vi "DetectorReadData-nil.vi"(8 "error in (no error)":errorcluster, 9 "disable averaging":bool, 10 "show flyback data":bool, 11 "Microscope in":refnum<class "Microscope.lvclass">) -> (0 "error out":errorcluster, 2 "Data":dbl[][](array[numeric]), 3 "Microscope out":refnum<class "Microscope.lvclass">)   [LabVIEW 2012, in "Microscope.lvclass"]
uses:
  classes/Microscope.lvclass
  classes/Microscope.lvclass/Microscope.ctl
  <resource>/objmgr/daqmx.rc
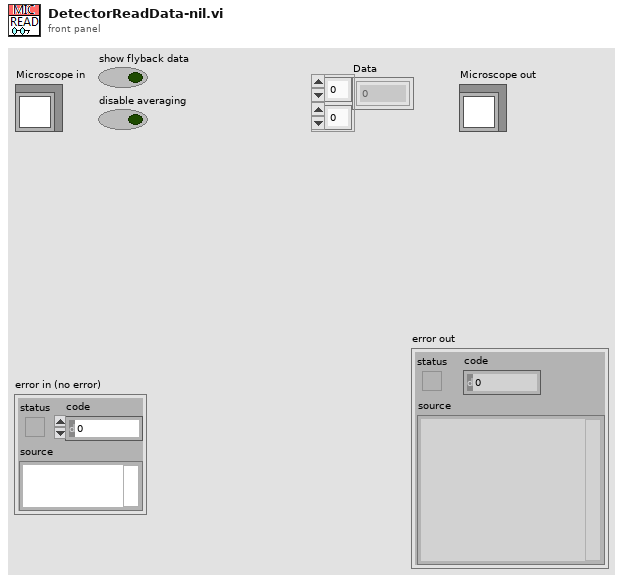
[diagram p1: front panel]
types:
  T1 = typedef "DetectorType.ctl" = enum16{"PMT", "SpectraWiz"}
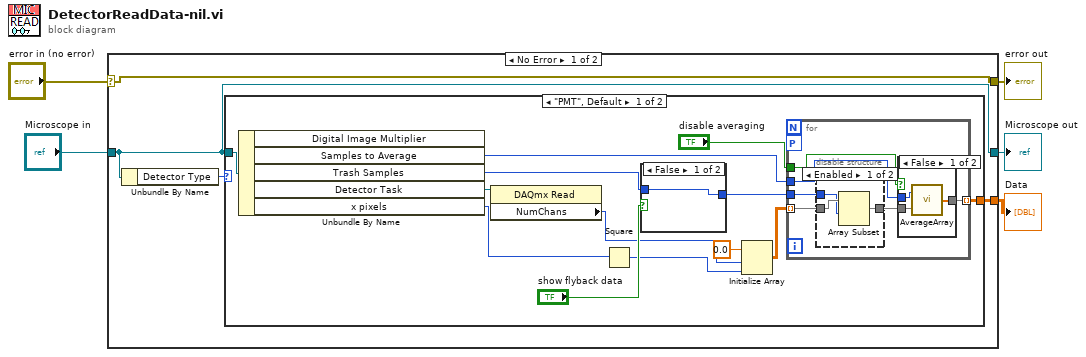
[diagram p0: block diagram]
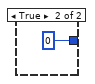
[diagram p2: hidden frame]
diagram:
  n1 = case shown="No Error" "error in (no error)" {
    selector: "error in (no error)" -> [w8 w40]
    tunnel: [w8 w40] -> w4
    tunnel: [w6 w39] -> w2
    tunnel: "Microscope in" -> [w6 w39]
    tunnel: [w9 _] -> w1
    frame No Error {
      n2 = Unbundle By Name(w6) -> ("Detector Type"=w7:T1)
      n3 = case shown="\"PMT\", Default" w7 {
        tunnel: [w22 _] -> w9
        tunnel: w6 -> [w10 _]
        frame "PMT", Default {
          n4 = Unbundle By Name(w10) -> ("Samples to Average"=w21:i32, "Trash Samples"=w20:i32, "Detector Task"=w15:refnum<k21>, "x pixels"=w13:i32)  [unwired: 1 out]
          n5 = property class="DAQmx Read"(reference=w15) -> ("NumChans"=w14:u32)  [unwired: 1 in, 2 out]
          n6 = Square(x=w13) -> (x^2=w12:i32)
          n7 = case shown="False" "show flyback data" {
            tunnel: w20 -> [w23 _]
            tunnel: [w23 0 ("Trash Samples")] -> w19
            frame False {
            }
            frame True {
            }
          }
          n8 = Initialize Array(0.0 ("element"), w14, w12) -> (w11:dbl[][])
          n9 = for {
            tunnel: w11 -> [w26] mode=indexing
            tunnel: w21 -> [w29]
            tunnel: w19 -> [w27]
            tunnel: [w28] -> w22 mode=indexing
            tunnel: "disable averaging" -> [w25]
            workers-P: _ -> [_]
            n10 = disable-structure shown="Enabled" {
              disable-tunnel: [w37 w38] -> w30
              disable-tunnel: w26 -> [w36 w38]
              disable-tunnel: w27 -> [w35 _]
              frame Enabled {
                n11 = Array Subset(array=w36, index=w35) -> (w37:dbl[])  [unwired: 1 in]
              }
              frame Disabled {
              }
            }
            n12 = case shown="False" w25 {
              tunnel: w30 -> [w33 w34]
              tunnel: w29 -> [w32 _]
              tunnel: [w31 w34] -> w28
              frame False {
                n13 = call "AverageArray.vi"("Input Array"=w33, "Samples To Average"=w32) -> ("Averaged Array"=w31:dbl[])
              }
              frame True {
              }
            }
          }
        }
        frame "SpectraWiz" {
        }
      }
    }
    frame Error {
    }
  }
  "error out" <- w4
  "Microscope out" <- w2
  "Data" <- w1
